vi "setSweep.vi"(4 "sweep type (0 : linear)":T1, 6 "Number of Points":i32, 8 "error in (no error)":errorcluster, 9 "Stop (Hz)":dbl, 10 "Start (Hz)":dbl, 11 "Instrument.VSource in":refnum<class "Instrument.VNA.lvclass">) -> (0 "error out":errorcluster, 3 "Instrument.VSource out":refnum<class "Instrument.VNA.lvclass">)   [LabVIEW 2019, in "Instrument.VNA.lvclass"]
uses:
  Instrument.VNA.lvclass
  Typedefs/Sweep Type--enum.ctl
  Typedefs/setSweep--cluster.ctl
  Typedefs/VNA.Commands--Enum.ctl
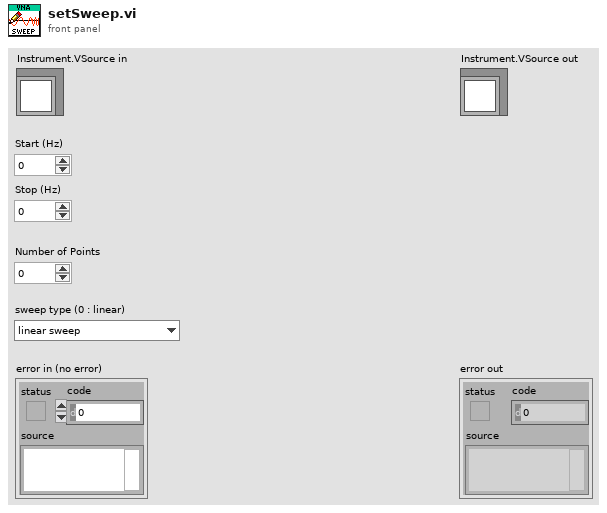
[diagram p1: front panel]
types:
  T1 = typedef "Instrument.VNA.lvclass/Sweep Type--enum.ctl" = enum16{"linear sweep", "logarithmic sweep", "frequency list", "CW time sweep", "power sweep"}
  T2 = typedef "Instrument.VNA.lvclass/VNA.Commands--Enum.ctl" = enum16{"getData", "setAverage", "setFormat", "setMeasurement", "setPower", "setSweep"}
  T3 = typedef "Instrument.VNA.lvclass/setSweep--cluster.ctl" = cluster{"start":dbl, "stop":dbl, "points":i32, "type":T1}
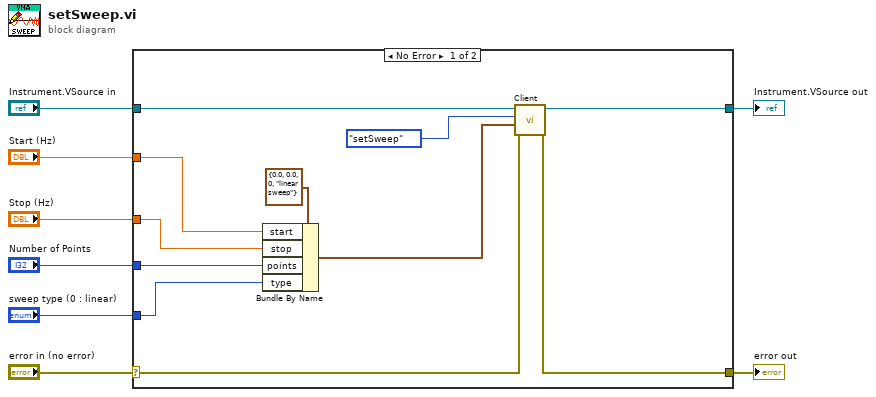
[diagram p0: block diagram]
diagram:
  n1 = case shown="No Error" "error in (no error)" {
    selector: "error in (no error)" -> [w10 w21]
    tunnel: [w18 w21] -> w7
    tunnel: [w19 w20] -> w5
    tunnel: "Instrument.VSource in" -> [w11 w20]
    tunnel: "Start (Hz)" -> [w13 _]
    tunnel: "Stop (Hz)" -> [w16 _]
    tunnel: "Number of Points" -> [w15 _]
    tunnel: "sweep type (0 : linear)" -> [w14 _]
    frame No Error {
      n2 = Bundle By Name(cluster=T3 {"start"=0.0, "stop"=0.0, "points"=0, "type"=enum."linear sweep"} ("setSweep"), "start"=w13, "stop"=w16, "points"=w15, "type"=w14) -> (w12:T3)
      n3 = call-dynamic "Client.vi"("error in (no error)"=w10, "Data in"=w12, "Command in"=VNA.Commands--Enum."setSweep" ("Commands"), "Instrument in"=w11) -> ("error out"=w18:errorcluster, "Instrument out"=w19:refnum<class "Instrument.VNA.lvclass">)  [unwired: 4 in, 2 out]
    }
    frame Error {
    }
  }
  "error out" <- w7
  "Instrument.VSource out" <- w5
